vi "proceed.vi"(8 "error in (no error)":errorcluster, 11 "GenericSweep in":refnum<class "GenericSweep.lvclass">) -> (0 "error out":errorcluster, 3 "GenericSweep out":refnum<class "GenericSweep.lvclass">)   [LabVIEW 2010, in "GenericSweep.lvclass"]
uses:
  GenericSweep.lvclass
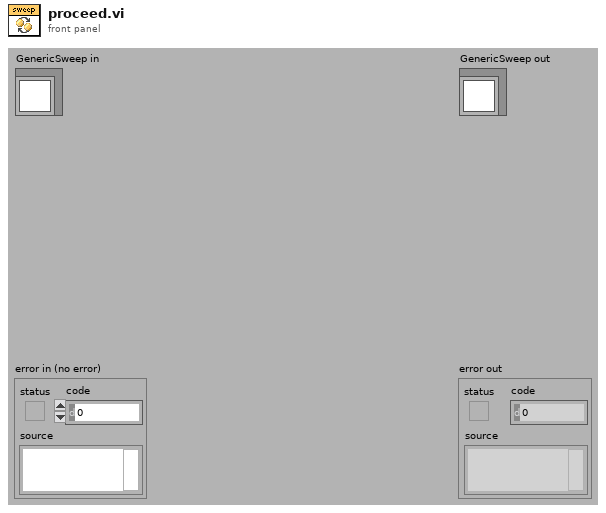
[diagram p1: front panel]
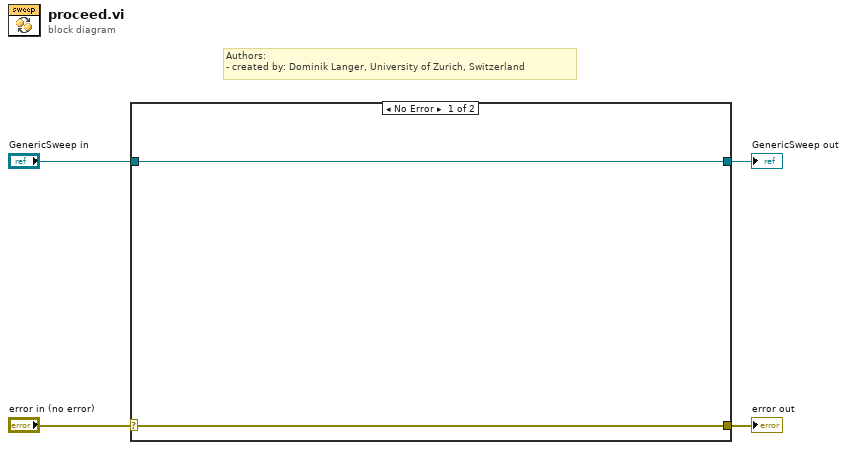
[diagram p0: block diagram]
diagram:
  # "Authors: \n- created by: Dominik Langer, University of Zurich, Switzerland"
  n1 = case shown="No Error" "error in (no error)" {
    selector: "error in (no error)" -> [w5 w8]
    tunnel: [w5 w8] -> w3
    tunnel: [w6 w7] -> w1
    tunnel: "GenericSweep in" -> [w6 w7]
    frame No Error {
    }
    frame Error {
    }
  }
  "error out" <- w3
  "GenericSweep out" <- w1
